vi "Create UA Server Tree.vi"(6 "Trusted Server Certificates":path[](array[path]), 7 "Username/Password":cluster{"Username":string, "Password":string}, 8 "Error In":errorcluster, 9 "Client Certificate File":path, 10 "Security Policy":T1, 11 "Server Endpoint URL":string) -> (0 "Error Out":errorcluster, 3 "UA Server Tree":refnum<class "UA Server.lvclass">)   [LabVIEW 2017, in "Browser Core.lvlib" / "UA Server.lvclass"]
doc: "Create OPC UA tree structure with root id. When the tree is created, a client connection to the OPC UA server will also be established."
uses:
  UA Server.lvclass
  C:/Users/MattJ/Desktop/GitHubSCM/UA-Server-Browser/source/Browser Core/Server Classes/Base Tree/Base Tree.lvclass
  UA Server.lvclass/UA Server.ctl
  <vilib>/OPCUA/NI OPC UA Client.lvlib
  Base Tree/Base Tree.lvclass
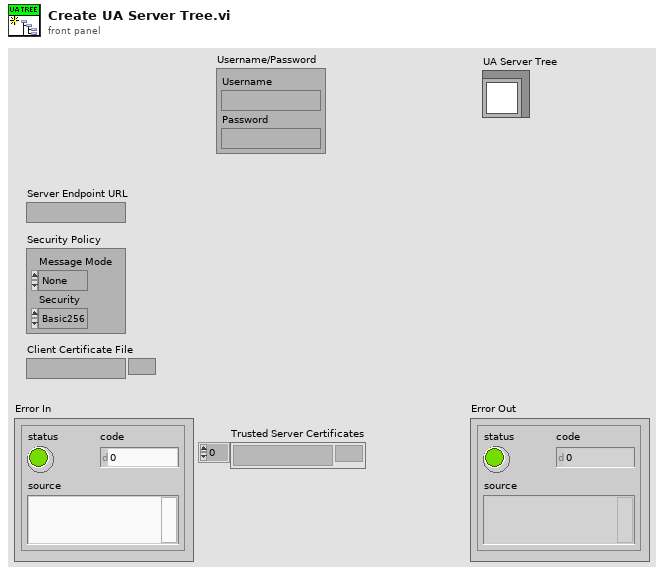
[diagram p1: front panel]
types:
  T1 = cluster{"Message Mode":enum16{"None", "Sign", "Sign and Encrypt"}, "Security":enum16{"Basic256", "Basic128Rsa15"}}
  T2 = typedef "OPC UA Client Refnum.ctl" = refnum<k21>
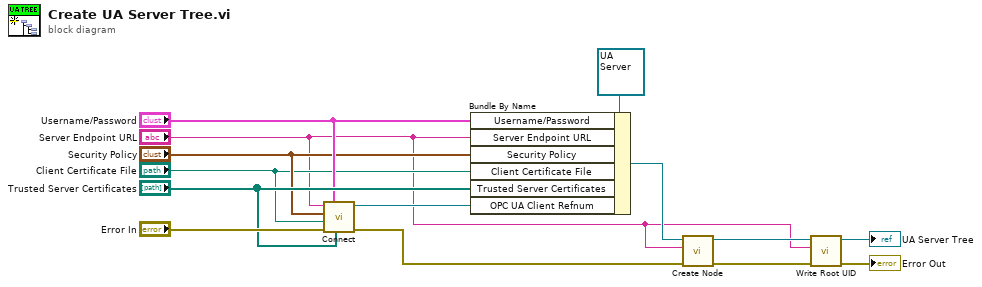
[diagram p0: block diagram]
diagram:
  n1 = call <vilib>:"Connect.vi"("trusted server certificates"="Trusted Server Certificates", "username/password"="Username/Password", "error in (no error)"="Error In", "client certificate file"="Client Certificate File", "security policy"="Security Policy", "server endpoint URL"="Server Endpoint URL") -> ("error out"=w6:errorcluster, "OPC UA client refnum out"=w12:T2)  [unwired: 3 in, 1 out]
  n2 = Bundle By Name(cluster=refnum<class "UA Server.lvclass"> refnum ("UA Server Tree"), "Username/Password"="Username/Password", "Server Endpoint URL"="Server Endpoint URL", "Security Policy"="Security Policy", "Client Certificate File"="Client Certificate File", "Trusted Server Certificates"="Trusted Server Certificates", "OPC UA Client Refnum"=w12) -> (w7:refnum<class "UA Server.lvclass">)
  n3 = call "Create Node.vi"("error in (no error)"=w6, "UID"="Server Endpoint URL", "Base Tree in"=w7) -> ("error out"=w5:errorcluster, "Base Tree out"=w4:refnum<class "UA Server.lvclass">)  [unwired: 7 in]
  n4 = call "Write Root UID.vi"("error in (no error)"=w5, "Root UID"="Server Endpoint URL", "Base Tree in"=w4) -> ("error out"=→"Error Out":errorcluster, "Base Tree out"=→"UA Server Tree":refnum<class "UA Server.lvclass">)  [unwired: 7 in]
